vi "Moving_Avg.vi"(10 "Num_Avg":dbl, 11 "Numeric in":dbl) -> (3 "Numeric out":dbl)   [LabVIEW 2015]
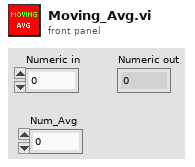
[diagram p1: front panel]
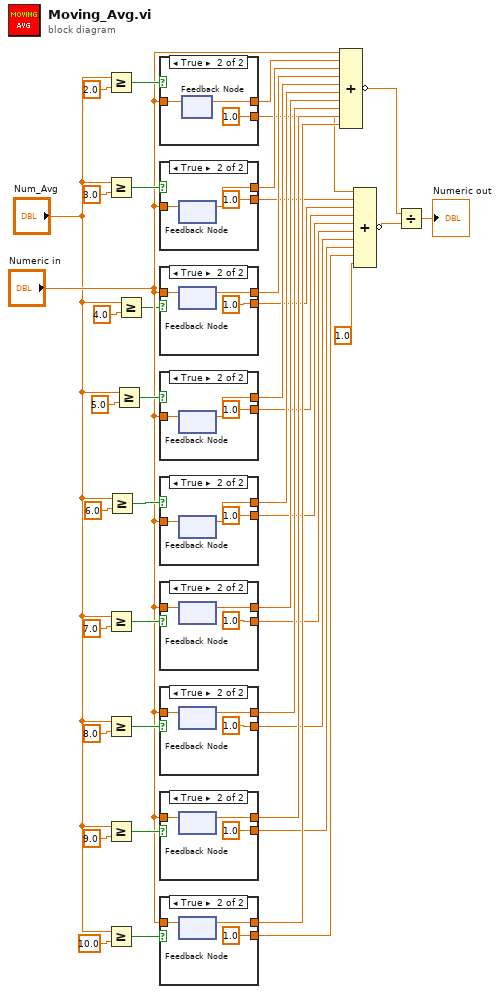
[diagram p0: block diagram]
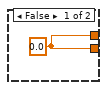
[diagram p2: hidden frame]
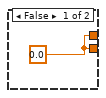
[diagram p3: hidden frame]
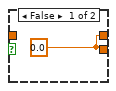
[diagram p4: hidden frame]
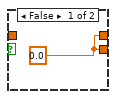
[diagram p5: hidden frame]
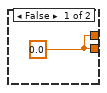
[diagram p6: hidden frame]
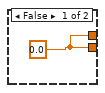
[diagram p7: hidden frame]
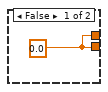
[diagram p8: hidden frame]
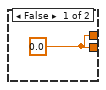
[diagram p9: hidden frame]
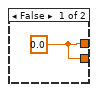
[diagram p10: hidden frame]
diagram:
  n1 = Greater Or Equal?(x="Num_Avg", y=2.0) -> (x >= y?=w41:bool)
  n2 = Greater Or Equal?(x="Num_Avg", y=3.0) -> (x >= y?=w40:bool)
  n3 = Greater Or Equal?(x="Num_Avg", y=7.0) -> (x >= y?=w37:bool)
  n4 = Greater Or Equal?(x="Num_Avg", y=8.0) -> (x >= y?=w36:bool)
  n5 = Greater Or Equal?(x="Num_Avg", y=9.0) -> (x >= y?=w35:bool)
  n6 = Greater Or Equal?(x="Num_Avg", y=10.0) -> (x >= y?=w34:bool)
  n7 = Greater Or Equal?(x="Num_Avg", y=6.0) -> (x >= y?=w38:bool)
  n8 = Greater Or Equal?(x="Num_Avg", y=5.0) -> (x >= y?=w39:bool)
  n9 = Greater Or Equal?(x="Num_Avg", y=4.0) -> (x >= y?=w2:bool)
  n10 = case shown="True" w41 {
    tunnel: "Numeric in" -> [_ w46]
    tunnel: [w43 w45] -> w25
    tunnel: [w43 1.0] -> w16
    frame False {
      w43 = 0.0
    }
    frame True {
      n11 = feedback #1() -> (w45:dbl)  [unwired: 1 in]
      n12 = feedback-in #1(w46) -> ()
    }
  }
  n13 = case shown="True" w40 {
    tunnel: "Numeric in" -> [_ w50]
    tunnel: [w47 w49] -> w24
    tunnel: [w47 1.0] -> w15
    frame False {
      w47 = 0.0
    }
    frame True {
      n14 = feedback #2() -> (w49:dbl)  [unwired: 1 in]
      n15 = feedback-in #2(w50) -> ()
    }
  }
  n16 = case shown="True" w2 {
    tunnel: "Numeric in" -> [_ w54]
    tunnel: [w51 w53] -> w23
    tunnel: [w51 1.0] -> w14
    frame False {
      w51 = 0.0
    }
    frame True {
      n17 = feedback #3() -> (w53:dbl)  [unwired: 1 in]
      n18 = feedback-in #3(w54) -> ()
    }
  }
  n19 = case shown="True" w39 {
    tunnel: "Numeric in" -> [_ w58]
    tunnel: [w55 w57] -> w22
    tunnel: [w55 1.0] -> w13
    frame False {
      w55 = 0.0
    }
    frame True {
      n20 = feedback #4() -> (w57:dbl)  [unwired: 1 in]
      n21 = feedback-in #4(w58) -> ()
    }
  }
  n22 = case shown="True" w38 {
    tunnel: "Numeric in" -> [_ w62]
    tunnel: [w59 w61] -> w21
    tunnel: [w59 1.0] -> w12
    frame False {
      w59 = 0.0
    }
    frame True {
      n23 = feedback #5() -> (w61:dbl)  [unwired: 1 in]
      n24 = feedback-in #5(w62) -> ()
    }
  }
  n25 = case shown="True" w37 {
    tunnel: "Numeric in" -> [_ w66]
    tunnel: [w63 w65] -> w20
    tunnel: [w63 1.0] -> w11
    frame False {
      w63 = 0.0
    }
    frame True {
      n26 = feedback #6() -> (w65:dbl)  [unwired: 1 in]
      n27 = feedback-in #6(w66) -> ()
    }
  }
  n28 = case shown="True" w36 {
    tunnel: "Numeric in" -> [_ w70]
    tunnel: [w67 w69] -> w19
    tunnel: [w67 1.0] -> w10
    frame False {
      w67 = 0.0
    }
    frame True {
      n29 = feedback #7() -> (w69:dbl)  [unwired: 1 in]
      n30 = feedback-in #7(w70) -> ()
    }
  }
  n31 = case shown="True" w35 {
    tunnel: "Numeric in" -> [_ w74]
    tunnel: [w71 w73] -> w18
    tunnel: [w71 1.0] -> w9
    frame False {
      w71 = 0.0
    }
    frame True {
      n32 = feedback #8() -> (w73:dbl)  [unwired: 1 in]
      n33 = feedback-in #8(w74) -> ()
    }
  }
  n34 = case shown="True" w34 {
    tunnel: "Numeric in" -> [_ w78]
    tunnel: [w75 w77] -> w17
    tunnel: [w75 1.0] -> w8
    frame False {
      w75 = 0.0
    }
    frame True {
      n35 = feedback #9() -> (w77:dbl)  [unwired: 1 in]
      n36 = feedback-in #9(w78) -> ()
    }
  }
  n37 = Compound Arithmetic op=ADD("Numeric in", w25, w24, w23, w22, w21, w20, w19, w18, w17) -> (invert w42:dbl)
  n38 = Compound Arithmetic op=ADD(w16, w15, w14, w13, w12, w11, w10, w9, w8, 1.0) -> (invert w7:dbl)
  n39 = Divide(x=w42, y=w7) -> (x/y=→"Numeric out":dbl)
